vi "Get Check Statement.vi"(8 "error in (no error)":errorcluster, 9 "Column Name Array":string[](array[string]), 10 "Table Name":string, 11 "MS Access in":refnum<class "MS Access.lvclass">) -> (0 "error out":errorcluster, 2 "Check Constraint Array":T1(array[cluster]), 3 "MS Access out":refnum<class "MS Access.lvclass">)   [LabVIEW 2020, in "MS Access.lvclass"]
uses:
  MS Access.lvclass
  ODBC/ADODB.lvclass
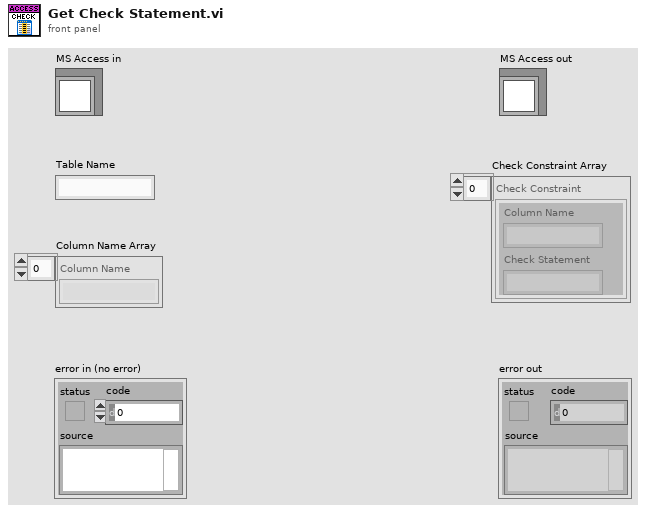
[diagram p1: front panel]
types:
  T1 = cluster{"Column Name":string, "Check Statement":string}[]
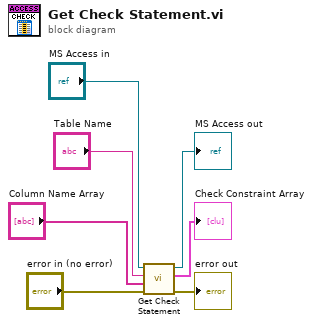
[diagram p0: block diagram]
diagram:
  n1 = call-parent "Get Check Statement.vi"("error in (no error)"="error in (no error)", "Column Name Array"="Column Name Array", "Table Name"="Table Name", "Database in"="MS Access in") -> ("error out"=→"error out":errorcluster, "Check Constraint Array"=→"Check Constraint Array":T1, "Database out"=→"MS Access out":refnum<class "MS Access.lvclass">)  [unwired: 5 in]
